vi "Time Estimate.vi"(8 "error in (no error)":errorcluster, 9 "expmode":i32, 10 "scantype":T1(ring), 11 "Varian Magnet Scan.lvclass":refnum<class "Varian Magnet Scan.lvclass">) -> (0 "error out":errorcluster, 1 "Time Estimate":string, 2 "time":dbl[unit], 3 "Varian Magnet Scan.lvclass out":refnum<class "Varian Magnet Scan.lvclass">)   [LabVIEW 2009, in "Varian Magnet Scan.lvclass"]
doc: "(Dynamic) Return an estimate of the time remaining to scan over this Scanner's preconfigured Range."
uses:
  Varian Magnet Scan.lvclass
  Scanner/Scanner.lvclass
  Scanner/Setup UI.vi
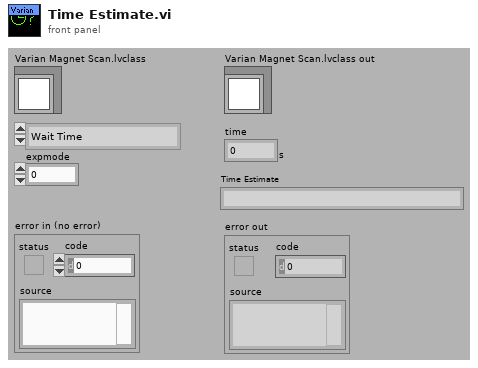
[diagram p1: front panel]
types:
  T1 = enum16{"Wait Time", "Pulse Width", "Wavelength", "Magnetic Field", "rf Scan"}
  T2 = typedef "Scanner.lvclass/Range.ctl" = cluster{"xi":dbl, "xf":dbl, "dx":dbl, "Return to...?":bool, "Return to":dbl}
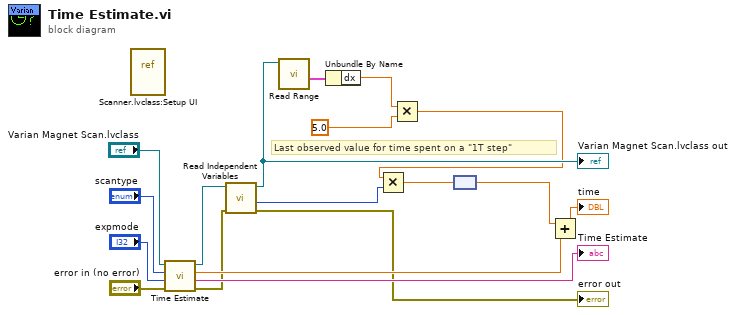
[diagram p0: block diagram]
diagram:
  # "Last observed value for time spent on a \"1T step\""
  n1 = vi-ref "Scanner.lvclass:Setup UI.vi"() -> ()  [unwired: 1 out]
  n2 = call-parent "Time Estimate.vi"("error in (no error)"="error in (no error)", "expmode"="expmode", "scantype"="scantype", "Scanner.lvclass"="Varian Magnet Scan.lvclass") -> ("error out"=w10:errorcluster, "Time Estimate"=→"Time Estimate":string, "time"=w17:dbl[unit], "Scanner.lvclass out"=w11:refnum<class "Varian Magnet Scan.lvclass">)  [unwired: 4 in]
  n3 = call-dynamic "Read Independent Variables.vi"("error in (no error)"=w10, "Scanner.lvclass in"=w11) -> ("error out"=→"error out":errorcluster, "size"=w8:i32, "Scanner.lvclass out"=w5:refnum<class "Varian Magnet Scan.lvclass">)  [unwired: 7 out]
  "Varian Magnet Scan.lvclass out" <- w5
  n4 = call-dynamic "Read Range.vi"("Scanner.lvclass in"=w5) -> ("Range"=w4:T2)  [unwired: 5 in, 5 out]
  n5 = Unbundle By Name(w4) -> ("dx"=w3:dbl)
  n6 = Multiply(x=w3, y=5.0) -> (x*y=w1:dbl)
  n7 = Multiply(x=w1, y=w8) -> (x*y=w7:dbl)
  n8 = node(w7) -> (w6:dbl[unit])
  n9 = Add(x=w6, y=w17) -> (x+y=→"time":dbl[unit])
